vi "TagBus_TEST_List All Tags.vi"(8 "error in (no error)":errorcluster, 11 "TagBus in":refnum<class "TagBus.lvclass">) -> (0 "error out":errorcluster, 1 "values":dbl[](array[numeric]), 2 "Double":string[](array[string]), 3 "TagBus out":refnum<class "TagBus.lvclass">)   [LabVIEW 2015, in "TagBus.lvclass"]
uses:
  TagBus.lvclass
  TagBus.lvclass/TagBus.ctl
  <vilib>/NI/Tag Bus/tag/Data Type.ctl
  <vilib>/NI/Tag Bus/table/data polymorphs/read many/read Doubles.vi
  <vilib>/NI/Tag Bus/dictionary/data dictionary.lvclass
  <vilib>/NI/Tag Bus/table/data table.lvlib
  <vilib>/NI/Tag Bus/tag/tag descriptor.lvclass
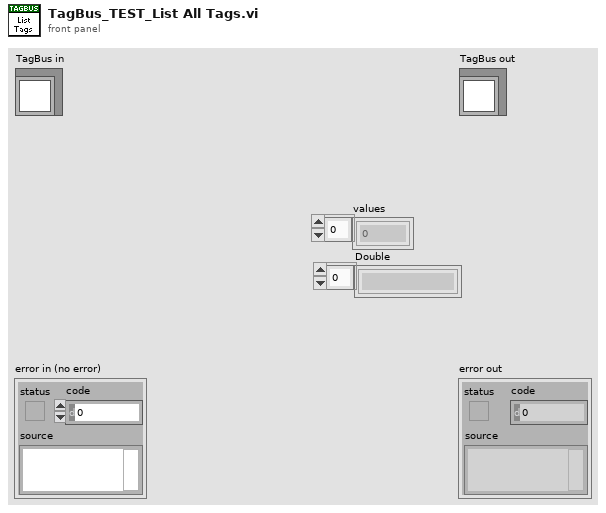
[diagram p1: front panel]
types:
  T1 = typedef "tag bus.lvlib/data table.lvlib/data table.ctl" = cluster{"Double":dbl[], "Single":sgl[], "I64":i64[], "I32":i32[], "I16":i16[], "I8":i8[], "U64":u64[], "U32":u32[], "U16":u16[], "U8":u8[], "Boolean":bool[], "String":string[], "Array of Double":cluster{"DBL Array":dbl[]}[], "Array of Single":cluster{"SGL Array":sgl[]}[], "Array of I64":cluster{"I64 Array":i64[]}[], "Array of I32":cluster{"I32 Array":i32[]}[], "Array of I16":cluster{"I16 Array":i16[]}[], "Array of I8":cluster{"I8 Array":i8[]}[], "Array of U64":cluster{"U64 Array":u64[]}[], "Array of U32":cluster{"U32 Array":u32[]}[], "Array of U16":cluster{"U16 Array":u16[]}[], "Array of U8":cluster{"U8 Array":u8[]}[], "Array of Boolean":cluster{"Boolean Array":bool[]}[], "Array of String":cluster{"String Array":string[]}[]}
  T2 = typedef "tag bus.lvlib/data dictionary.lvclass/full data dictionary.ctl" = cluster{"Double":string[], "Single":string[], "I64":string[], "I32":string[], "I16":string[], "I8":string[], "U64":string[], "U32":string[], "U16":string[], "U8":string[], "Boolean":string[], "String":string[], "Array of Double":string[], "Array of Single":string[], "Array of I64":string[], "Array of I32":string[], "Array of I16":string[], "Array of I8":string[], "Array of U64":string[], "Array of U32":string[], "Array of U16":string[], "Array of U8":string[], "Array of Boolean":string[], "Array of String":string[]}
  T3 = typedef "tag bus.lvlib/tag descriptor.lvclass/Data Type.ctl" = enum16{"Double", "Single", "I64", "I32", "I16", "I8", "U64", "U32", "U16", "U8", "Boolean", "String", "Array of Double", "Array of Single", "Array of I64", "Array of I32", "Array of I16", "Array of I8", "Array of U64", "Array of U32", "Array of U16", "Array of U8", "Array of Boolean", "Array of String"}
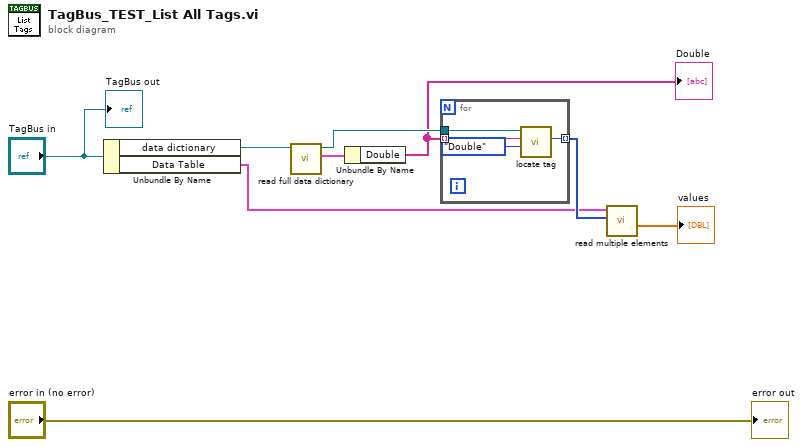
[diagram p0: block diagram]
diagram:
  n1 = Unbundle By Name("TagBus in") -> ("data dictionary"=w8:refnum<class "data dictionary.lvclass">, "Data Table"=w3:T1)
  n2 = call <vilib>:"read full data dictionary.vi"("data dictionary in"=w8) -> ("dictionary"=w7:T2, "data dictionary out"=w6:refnum<class "data dictionary.lvclass">)  [unwired: 8 in, 1 out]
  n3 = Unbundle By Name(w7) -> ("Double"=w5:string[])
  "Double" <- w5
  n4 = for {
    tunnel: w6 -> [w13]
    tunnel: w5 -> [w12] mode=indexing
    tunnel: [w10] -> w4 mode=indexing
    n5 = call <vilib>:"locate tag.vi"("data type"=Data_Type."Double", "name"=w12, "data dictionary in"=w13) -> ("index"=w10:i32)  [unwired: 6 in, 2 out]
  }
  n6 = call-poly <vilib>:"read multiple elements.vi"("indices"=w4, "data table in"=w3) -> ("values"=→"values":dbl[])  [unwired: 8 in, 1 out]
  "error out" <- "error in (no error)"
  "TagBus out" <- "TagBus in"
